vi "JKI_DataBase.vi"() -> ()   [LabVIEW 2017, in "Database.lvlib"]
uses:
  Database.lvlib
  <userlib>/_NEVSTOP/JKI State Machine ++/_Support/_Create Data Queue.vi
  <vilib>/Utility/file.llb/Read Delimited Spreadsheet (string).vi
  <userlib>/_NEVSTOP/JKI State Machine ++/_Support/_JKISMQFGV.vi
  <vilib>/Utility/file.llb/Write Delimited Spreadsheet (string).vi
  <userlib>/_NEVSTOP/JKI State Machine ++/JKI-State-Machine-Plus.lvlib
panel:
  in  "Error Simulator":bool
  out "Balance":i32
  out "Find Account?":bool
  in  "Get Balance Simulator":bool
  in  "Update Simulator":bool
  in  "Find Account Simulator":bool
  out "若有需要返回用户姓名，后面也可以接到esponse上":string
  out "State History":string
  in  "Name(\"\" to use uuid)":string="Database"
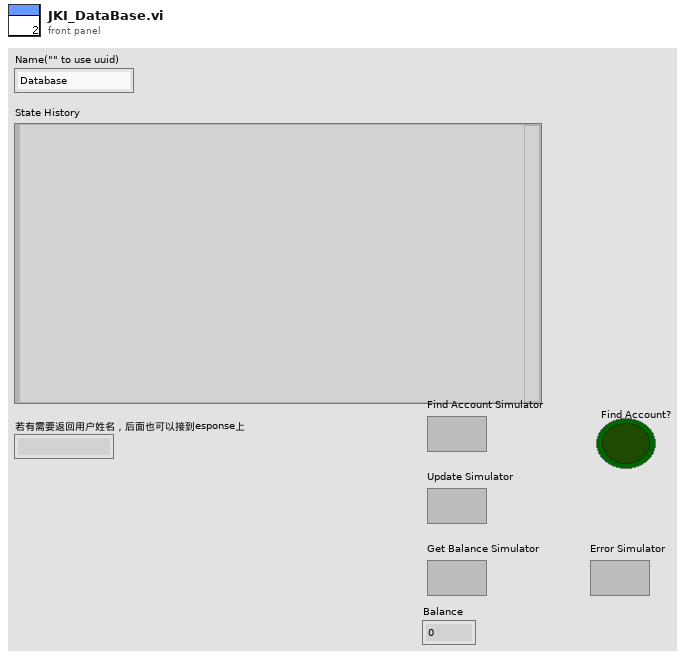
[diagram p1: front panel]
types:
  T1 = enum32{"Invalid", "Standard", "Closed", "Hidden", "Minimized", "Maximized"}
  T2 = enum32{"invalid app kind", "Development System", "Run Time System", "Student Edition", "Embedded LabVIEW", "Evaluation", "Custom"}
  T3 = cluster{"Core":cluster{"Current VI Reference":refnum<vi>, "Close Panel on Exit?":bool}}
  T4 = cluster{"PIN":string, "First":string, "Last":string, "Amount":string}
  T5 = cluster{"Current VI Reference":refnum<vi>, "Close Panel on Exit?":bool}
  T6 = cluster{"PIN":string, "First":string, "Last":string, "Amount":string}[]
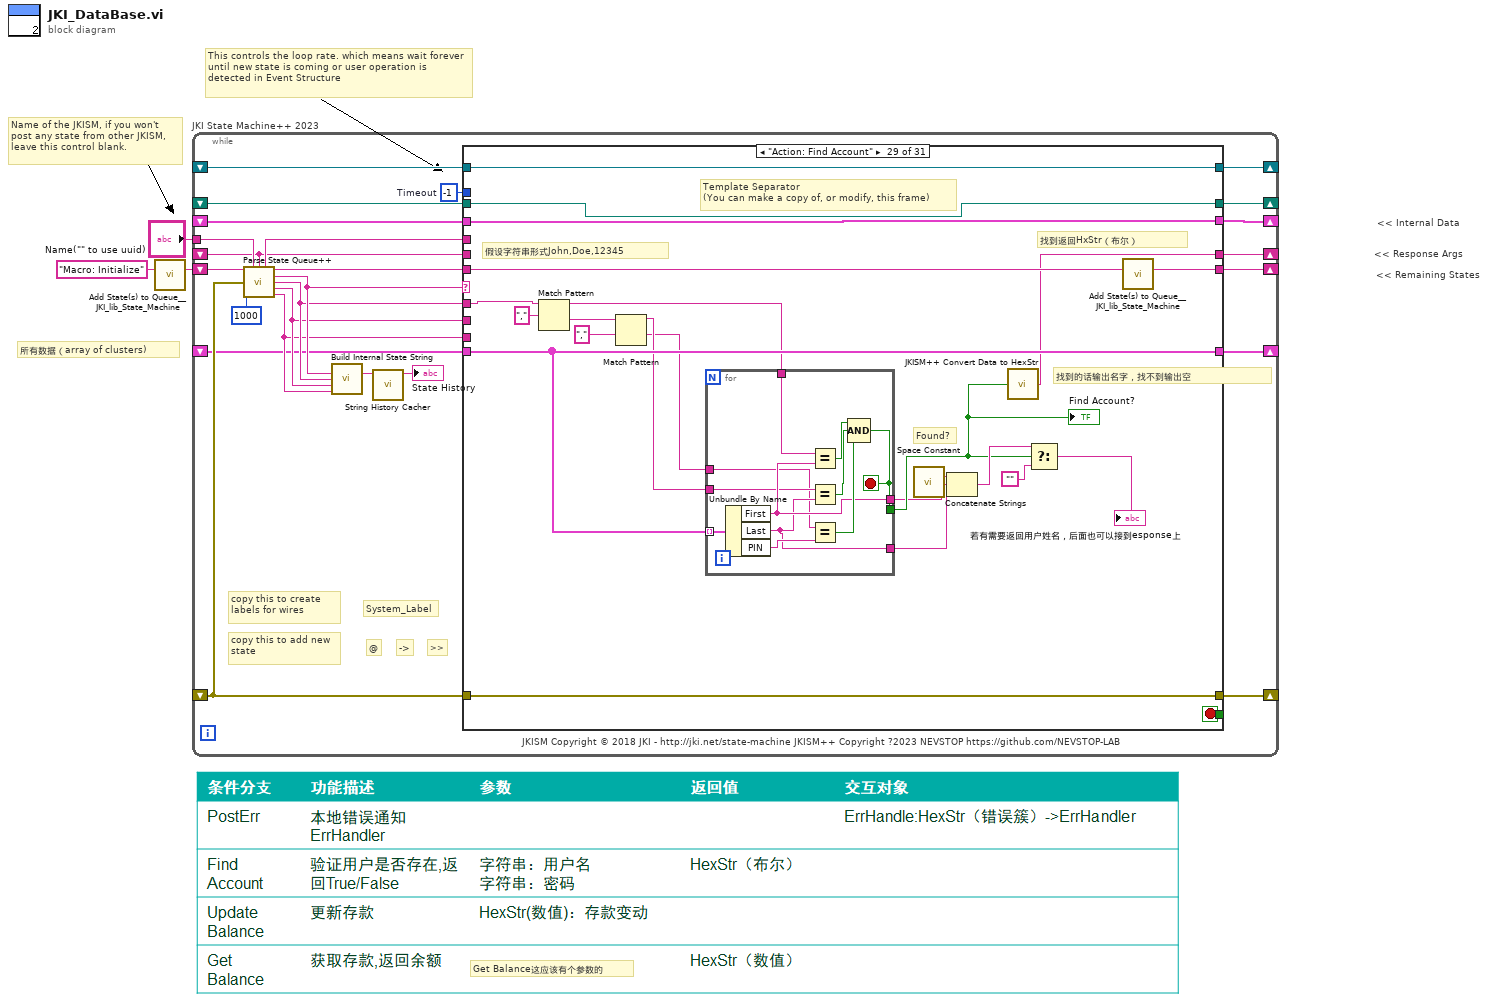
[diagram p0: block diagram]
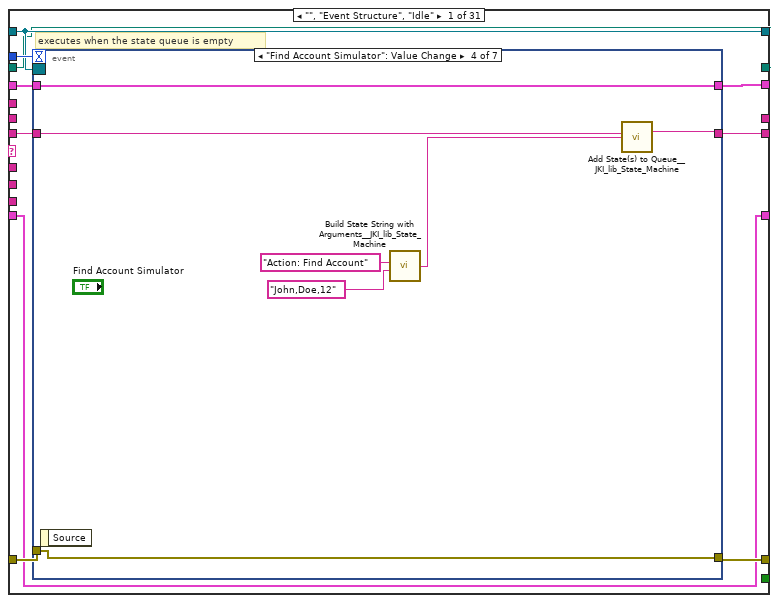
[diagram p2: hidden frame]
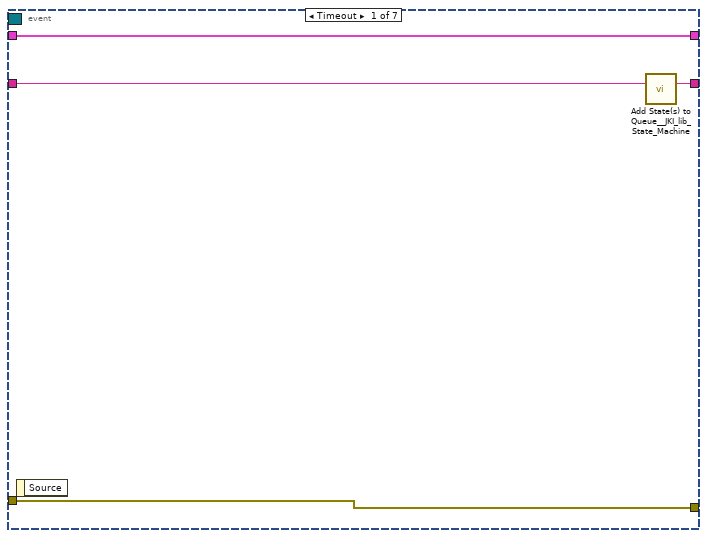
[diagram p3: hidden frame]
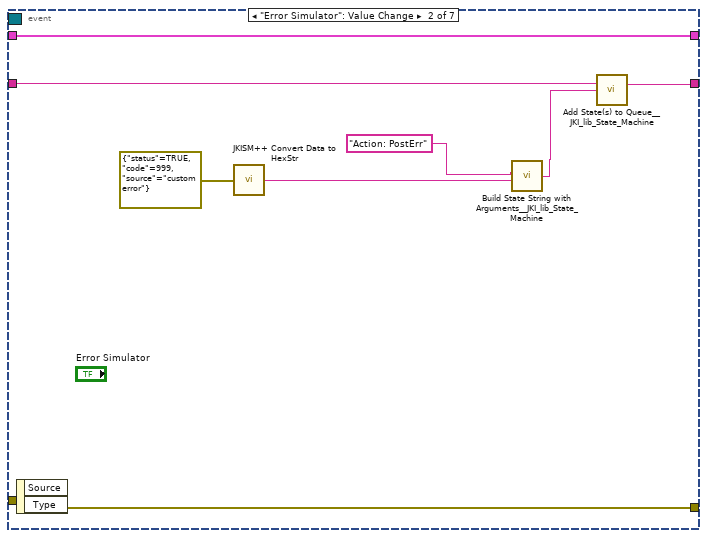
[diagram p4: hidden frame]
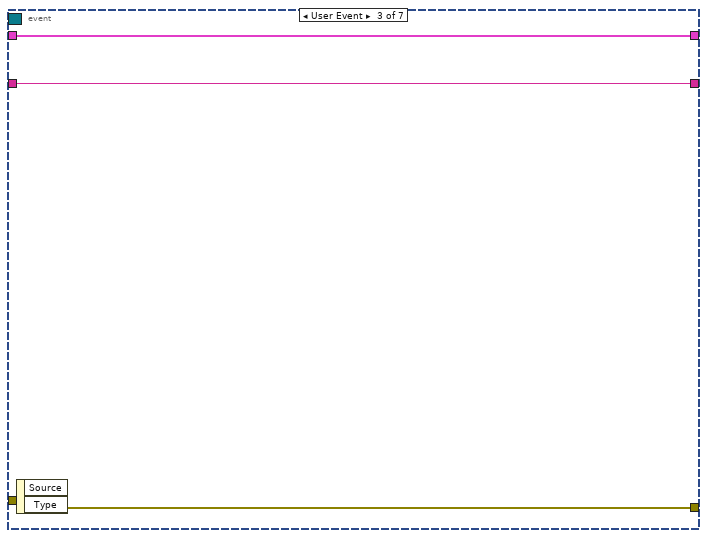
[diagram p5: hidden frame]
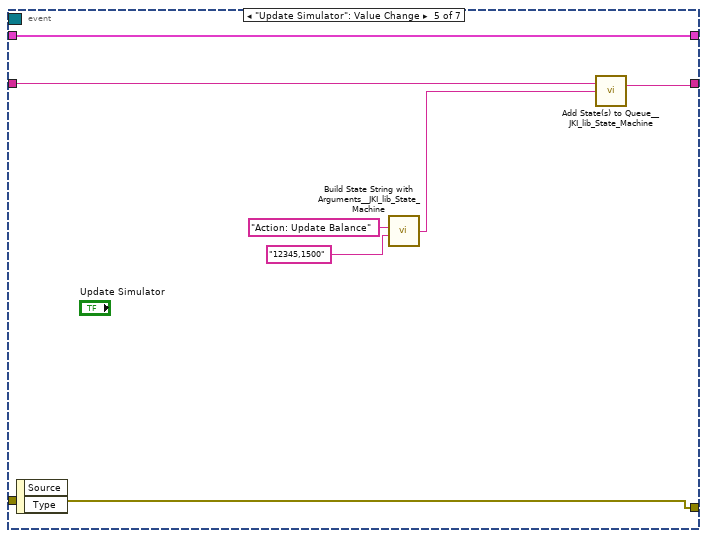
[diagram p6: hidden frame]
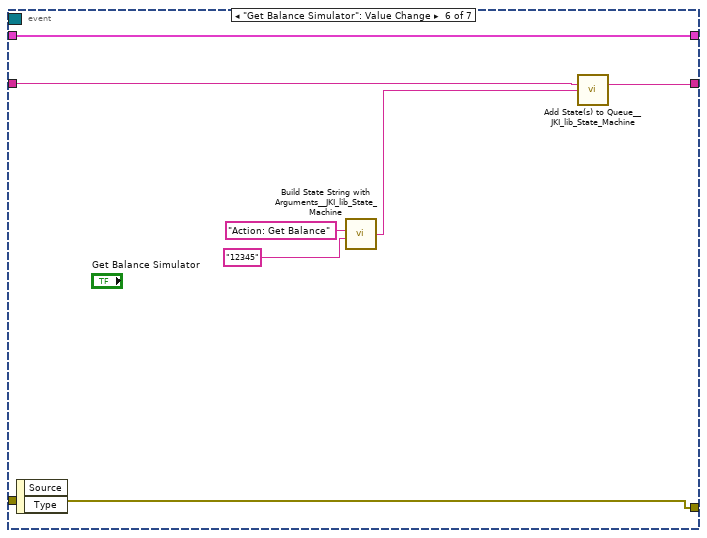
[diagram p7: hidden frame]
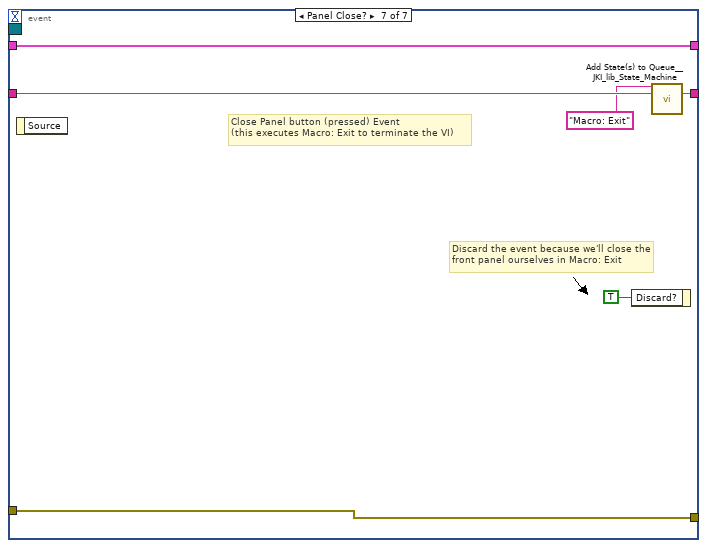
[diagram p8: hidden frame]
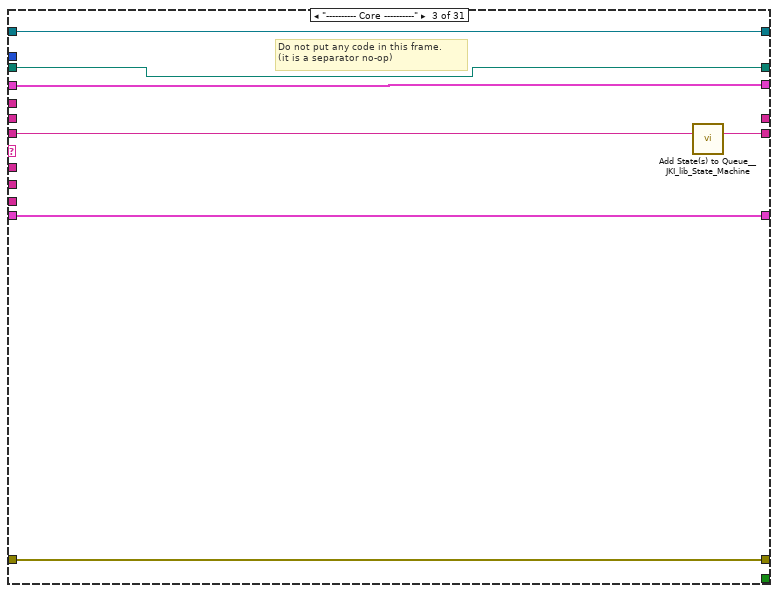
[diagram p10: hidden frame]
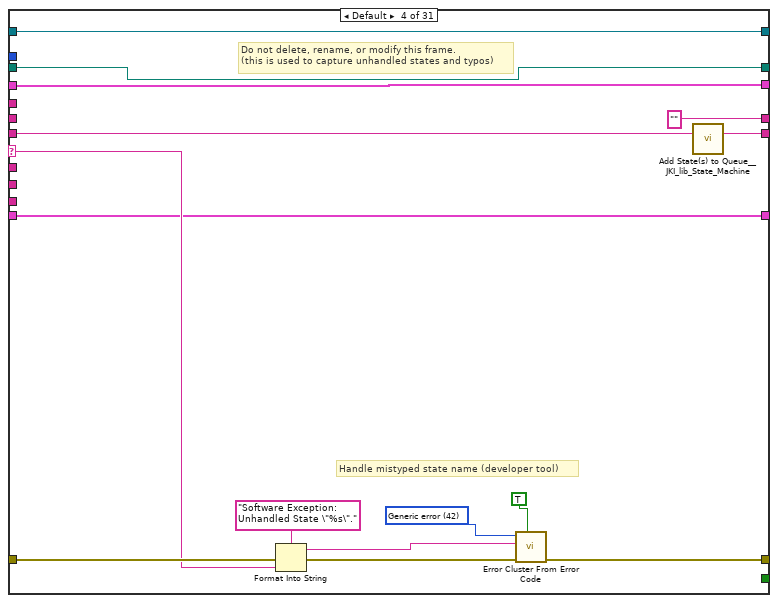
[diagram p11: hidden frame]
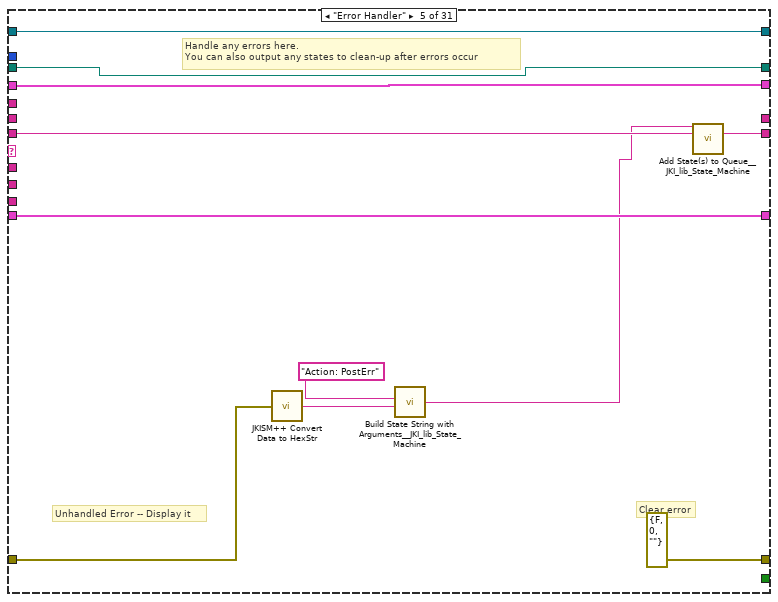
[diagram p12: hidden frame]
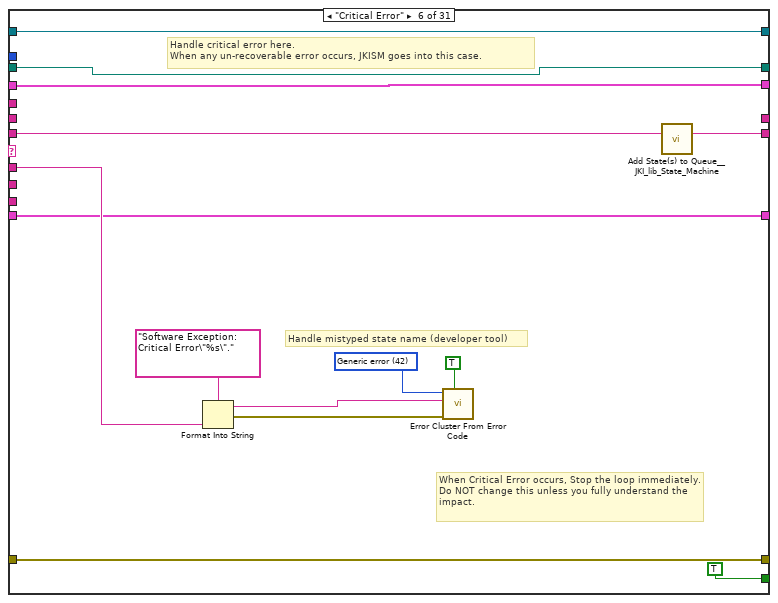
[diagram p13: hidden frame]
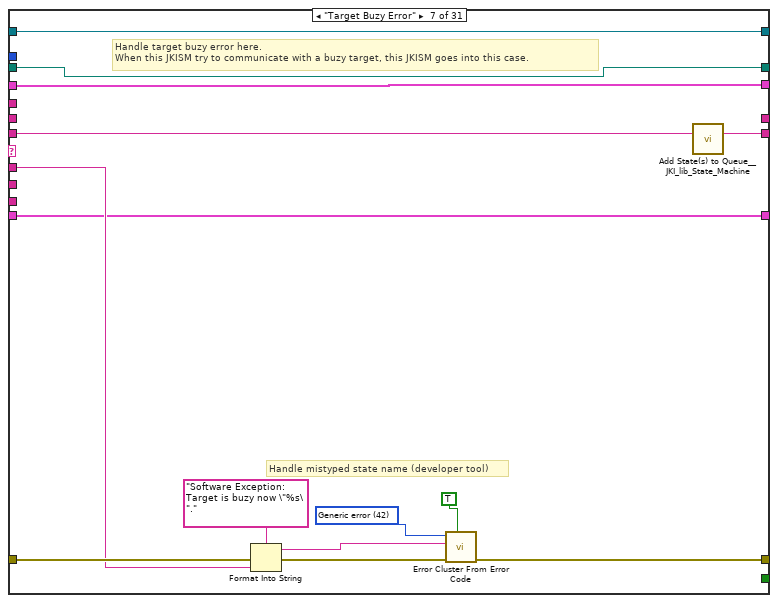
[diagram p14: hidden frame]
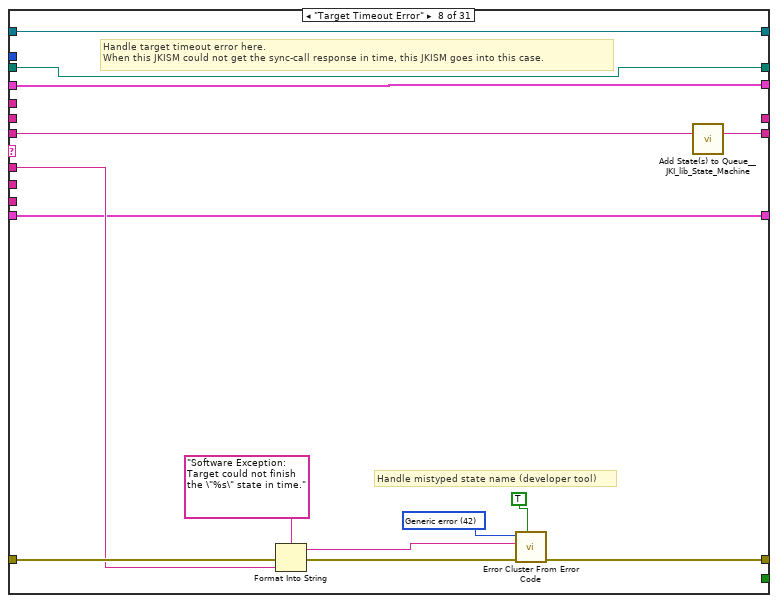
[diagram p15: hidden frame]
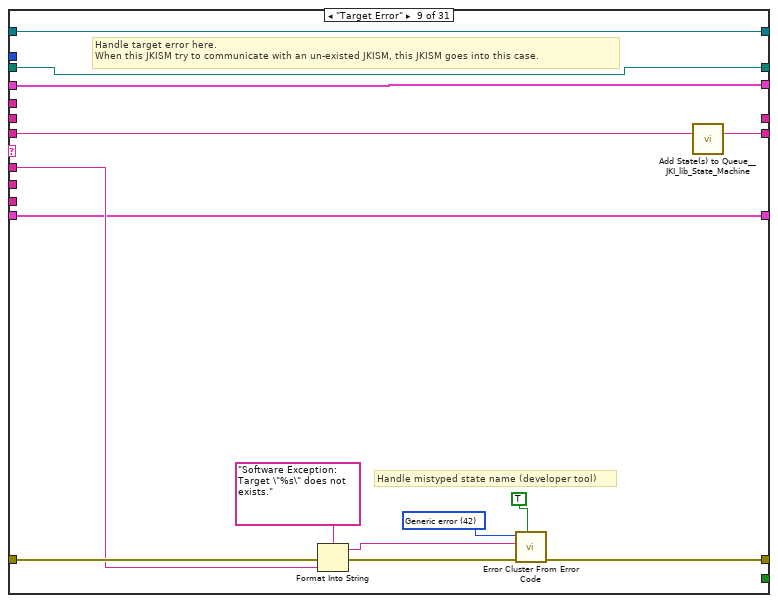
[diagram p16: hidden frame]
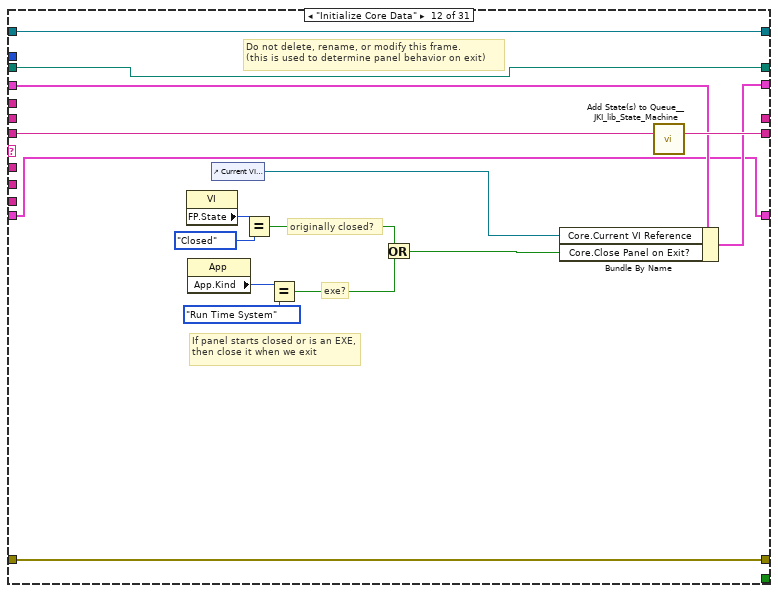
[diagram p19: hidden frame]
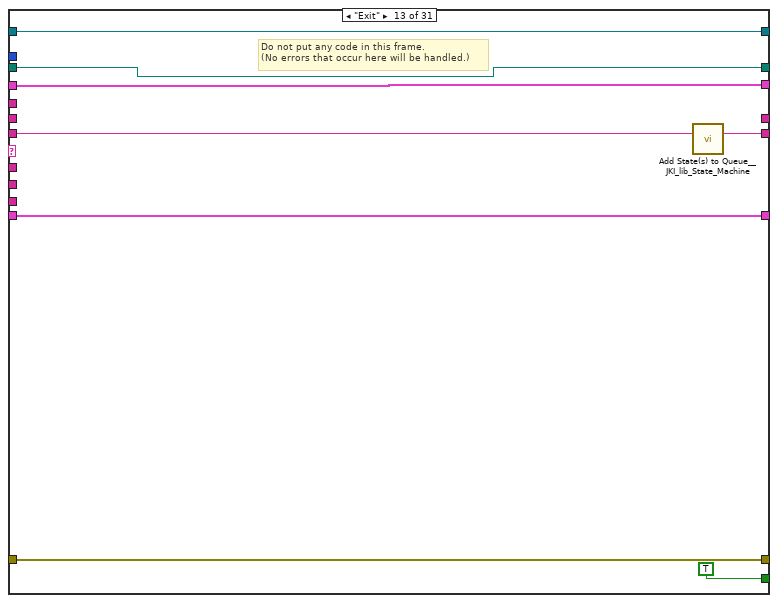
[diagram p20: hidden frame]
diagram:
  # "Get Balance这应该有个参数的"
  # "所有数据（array of clusters)"
  # "<< Internal Data"
  # "<< Response Args"
  # "<< Remaining States"
  # "Name of the JKISM, if you won't post any state from other JKISM,  leave this control blank."
  # "This controls the loop rate. which means wait forever until new state is coming or user operation is detected in Event Structure"
  n1 = call <vilib>:"Add State(s) to Queue__JKI_lib_State_Machine.vi"("State(s) in (\"\")"="Macro: Initialize") -> ("States Out"=w1:string)  [unwired: 14 in]
  n2 = while "JKI State Machine++ 2023" {
    shift-right: [w24] -> _
    shift-left: _ -> [w23]
    shift-right: [w27] -> _
    shift-left: _ -> [w21]
    shift-right: [w26] -> _
    shift-left: w1 -> [w28]
    tunnel: "Name(\"\" to use uuid)" -> [w16]
    shift-right: [w19] -> _
    shift-left: _ -> [w8]
    shift-right: [w18] -> _
    shift-left: _ -> [w17]
    shift-right: [w7] -> _
    shift-left: _ -> [w6]
    shift-right: [w5] -> _
    shift-left: _ -> [w4]
    stop <- w25 stop-if-true
    w22 = -1  # Timeout
    # "JKISM Copyright © 2018 JKI - http://jki.net/state-machine JKISM++ Copyright ?2023 NEVSTOP https://github.com/NEVSTOP-LAB"
    # "copy this to add new state"
    # ">>"
    # "->"
    # "@"
    # "copy this to create labels for wires"
    # "System_Label"
    n3 = call <userlib>:"Parse State Queue++.vi"("State Queue"=w28, "Name(\"\" to use uuid)"=w16, "Response Arguments"=w8, "Error In (no error)"=w21, "Response Timeout(5000ms)"=1000 ("Response Timeout(1000ms)")) -> ("Name Used"=w9:string, "Remaining States"=w29:string, "Current State"=w13:string, "Arguments"=w12:string, "Argument - State"=w11:string, "From Who"=w10:string)  [unwired: 5 in]
    n4 = call <userlib>:"Build Internal State String.vi"("State"=w13, "Arguments (\"\")"=w12, "Arg-State (\"\")"=w11, "Source (\"\")"=w10) -> ("State with Arguments"=w14:string)  [unwired: 11 in]
    n5 = call <userlib>:"String History Cacher.vi"("String"=w14) -> ("String Cache"=→"State History":string)  [unwired: 10 in]
    n6 = case shown="\"Action: Find Account\"" w13 {
      selector: w13 -> [_ _ _ w99 _ _ _ _ _ _ _ _ _ _ _ _ _ _ _ _ _ _ _ _ _ _ _ _ _ _ _]
      tunnel: w29 -> [w39 w86 w94 w103 w120 w132 w137 w156 w170 w181 w187 w204 w212 w219 w232 w248 w255 w263 w269 w277 w284 w293 w307 w374 w382 w395 w402 w410 w435 w474 w492]
      tunnel: w12 -> [_ _ _ _ _ w125 w139 w152 w166 _ _ _ _ _ _ _ _ _ _ _ _ w288 w302 _ _ _ _ w406 w428 w460 w485]
      tunnel: w23 -> [w37 w85 w91 w101 w117 w133 w141 w154 w168 w180 w186 w191 w210 w216 _ w242 w252 w262 w268 w274 w282 w291 w299 w371 w379 w385 w399 w414 w434 w472 w489]
      tunnel: [w36 w87 w92 w105 errorcluster {"status"=FALSE, "code"=0, "source"=""} ("error out") w134 w144 w158 w172 w182 w188 w202 w209 w217 w230 w245 w253 w258 w267 w275 w281 w289 w304 w372 w380 w393 w400 w404 w445 w461 w490] -> w27
      tunnel: w21 -> [w35 w87 w92 w104 w111 w134 w143 w157 w171 w182 w188 w202 w209 w217 w230 w246 w253 _ w270 w275 w281 w290 w305 w372 w380 w393 w400 w405 w445 _ w490]
      tunnel: [w38 w86 w93 w102 w119 w131 w142 w155 w169 w181 w187 w203 w211 w218 w231 w247 w254 w263 w269 w276 w283 w292 w306 w373 w381 w394 w401 w409 w436 w473 w491] -> w26
      tunnel: [_ _ _ _ _ TRUE _ _ _ _ _ _ TRUE _ _ _ _ _ _ _ _ _ _ _ _ _ _ _ _ _ _] -> w25
      tunnel: [w34 w85 w91 w101 w117 w133 w141 w154 w168 w180 w186 w190 w210 w216 w221 w242 w252 w262 w268 w274 w282 w291 w299 w371 w379 w385 w399 w414 w434 w472 w489] -> w24
      tunnel: w22 -> [w33 _ _ _ _ _ _ _ _ _ _ _ _ _ _ _ _ _ _ _ _ _ _ _ _ _ _ _ _ _ _]
      tunnel: w10 -> [_ _ _ _ _ _ _ _ _ _ _ _ _ _ _ _ _ _ _ _ _ _ _ _ _ _ _ _ _ _ _]
      tunnel: w11 -> [_ _ _ _ _ _ _ _ _ _ _ _ _ _ _ _ _ _ _ _ _ _ _ _ _ _ _ _ _ _ _]
      tunnel: [_ _ _ "" _ _ _ _ _ _ _ _ _ _ _ _ _ _ _ _ _ _ _ _ _ _ _ _ w424 _ w483] -> w19
      tunnel: [w32 w84 w90 w97 w116 w123 w138 w151 w165 w179 w185 w193 w207 w215 w228 w244 w251 w261 w266 w273 w280 w287 w301 w370 w377 w387 w398 w413 w444 w471 w488] -> w18
      tunnel: w17 -> [w32 w84 w90 w97 w116 w123 w138 w151 w165 w179 w185 w193 w207 w215 w228 w244 w251 _ w266 w273 w280 w287 w301 w370 w377 w387 w398 w413 w444 w471 w488]
      tunnel: w9 -> [_ _ _ _ _ _ _ _ _ _ _ _ _ _ _ _ _ w260 _ _ _ _ _ _ _ _ _ _ _ _ _]
      tunnel: w8 -> [_ _ _ _ _ _ _ _ _ _ _ _ _ _ _ _ _ _ _ _ _ _ _ _ _ _ _ _ _ _ _]
      tunnel: [w31 w83 w89 w96 w115 w122 w136 w150 w164 w178 w184 w192 w206 w214 w223 w243 w250 w257 w265 w272 w279 w286 w300 w369 w376 w386 w397 w412 w443 w463 w487] -> w7
      tunnel: w6 -> [w31 w83 w89 w96 w115 w122 w136 w150 w164 w178 w184 w192 w206 w214 _ w243 w250 w257 w265 w272 w279 w286 w300 w369 w376 w386 w397 w412 w443 w463 w487]
      tunnel: [w30 w82 w88 w95 w114 w121 w135 w149 w163 w177 w183 w189 w205 w213 w220 w240 w249 w256 w264 w271 w278 w285 w298 w368 w375 w383 w396 w411 w439 w462 w486] -> w5
      tunnel: w4 -> [w30 w82 w88 w95 w114 w121 w135 w149 w163 w177 w183 w189 w205 w213 _ w240 w249 w256 w264 w271 w278 w285 w298 w368 w375 w383 w396 w411 w439 w468 w486]
      frame "", "Event Structure", "Idle" {
        # "executes when the state queue is empty"
        n7 = event shown="[3] \"Find Account Simulator\": Value Change" {
          selector: w32 -> [_ _ _ _ _ _ _]
          dyn-events: _ -> [_ _ _ _ _ _ _]
          timeout: w33 -> [_ _ _ _ _ _ _]
          tunnel: w39 -> [w43 w46 w54 w59 w66 w71 w81]
          tunnel: [w42 w45 w54 w58 w65 w70 w80] -> w38
          tunnel: w37 -> [w40 w50 w52 w61 w68 w75 w78]
          tunnel: [w41 w51 w53 w60 w67 w74 w79] -> w36
          tunnel: w35 -> [w41 w51 w53 w60 w67 w74 w79]
          tunnel: [w40 w50 w52 w61 w68 w75 w78] -> w34
          event Timeout {
            n8 = event-data() -> ()  [unwired: 1 in, 1 out]
            n9 = call <vilib>:"Add State(s) to Queue__JKI_lib_State_Machine.vi"("State(s) in (\"\")"=w43) -> ("States Out"=w42:string)  [unwired: 14 in]
          }
          event "Error Simulator": Value Change {
            n10 = event-data() -> ()  [unwired: 1 in, 2 out]
            n11 = call <userlib>:"JKISM++ Convert Data to HexStr.vi"("Variant"=errorcluster {"status"=TRUE, "code"=999, "source"="custom error"} ("error in (no error)")) -> ("HEX String (0-9,A-F)"=w47:string)  [unwired: 8 in]
            n12 = call <vilib>:"Build State String with Arguments__JKI_lib_State_Machine.vi"("Arguments (\"\")"=w47, "State"="Action: PostErr" ("States")) -> ("State with Arguments"=w44:string)  [unwired: 4 in]
            n13 = call <vilib>:"Add State(s) to Queue__JKI_lib_State_Machine.vi"("State(s) in (\"\")"=w46, "State(s) at Back (\"\")"=w44) -> ("States Out"=w45:string)  [unwired: 13 in]
          }
          event User Event {
            n14 = event-data() -> ()  [unwired: 1 in, 2 out]
          }
          event "Find Account Simulator": Value Change {
            n15 = event-data() -> ()  [unwired: 1 in, 1 out]
            n16 = call <vilib>:"Build State String with Arguments__JKI_lib_State_Machine.vi"("Arguments (\"\")"="John,Doe,12", "State"="Action: Find Account") -> ("State with Arguments"=w55:string)  [unwired: 4 in]
            n17 = call <vilib>:"Add State(s) to Queue__JKI_lib_State_Machine.vi"("State(s) in (\"\")"=w59, "State(s) at Back (\"\")"=w55) -> ("States Out"=w58:string)  [unwired: 13 in]
          }
          event "Update Simulator": Value Change {
            n18 = event-data() -> ()  [unwired: 1 in, 2 out]
            n19 = call <vilib>:"Build State String with Arguments__JKI_lib_State_Machine.vi"("Arguments (\"\")"="12345,1500", "State"="Action: Update Balance") -> ("State with Arguments"=w62:string)  [unwired: 4 in]
            n20 = call <vilib>:"Add State(s) to Queue__JKI_lib_State_Machine.vi"("State(s) in (\"\")"=w66, "State(s) at Back (\"\")"=w62) -> ("States Out"=w65:string)  [unwired: 13 in]
          }
          event "Get Balance Simulator": Value Change {
            n21 = event-data() -> ()  [unwired: 1 in, 2 out]
            n22 = call <vilib>:"Build State String with Arguments__JKI_lib_State_Machine.vi"("Arguments (\"\")"="12345", "State"="Action: Get Balance") -> ("State with Arguments"=w69:string)  [unwired: 4 in]
            n23 = call <vilib>:"Add State(s) to Queue__JKI_lib_State_Machine.vi"("State(s) in (\"\")"=w71, "State(s) at Back (\"\")"=w69) -> ("States Out"=w70:string)  [unwired: 13 in]
          }
          event Panel Close? {
            # "Discard the event because we'll close the front panel ourselves in Macro: Exit"
            # "Close Panel button (pressed) Event\n(this executes Macro: Exit to terminate the VI)"
            n24 = event-data() -> ()  [unwired: 1 in, 1 out]
            n25 = event-data("Discard?"=TRUE) -> ()  [unwired: 1 in, 1 out]
            n26 = call <vilib>:"Add State(s) to Queue__JKI_lib_State_Machine.vi"("State(s) in Front (\"\")"="Macro: Exit", "State(s) in (\"\")"=w81) -> ("States Out"=w80:string)  [unwired: 13 in]
          }
        }
      }
      frame "JKISM++ Documentation" {
        # "JKISM++ Documentation"
        # "State Syntax:\nStateCategory: State >> Argument @|-> JKISMName\nLine Terminator: Line feed\n\nExample:\nUI: Help >> About @Main\nUI: Help >> About ->Main"
        # "Commenting:\nTo add a comment use \"//\" or \"#\" and all text to the right will be ignored\nCommenting Example:\nUI: Initialize // This initializes the UI\n# This whole line is a comment\n// Another comment line"
        # "Where \"UI\" is the state category\nWhere \"Help\" is the state\nWhere \"About\" is the argument\nWhere \"Main\" is the Name of JKISM,which actually run the \"UI: Help >> About\"\n\n    \"@\" stands for sync state. Current JKISM will wait until the state is finished. \n            - if \"Main\" named JKISM does not exist, \"Target Error\" will occur.\n            - if \"Main\" named JKISM is in another sync remote state, \"Target Buzy Error\" will occur.\n            - if \"Main\" named JKISM could not finish the state in time, \"Target Timeout Error\" will occur.\n            - if everything is right. \"Response\" will occur with Argument back from \"Main\" named JKISM. \n\n    \"->\" stands for async state. Current JKISM will post the state and continue to next state in next iteration.\n            - if \"Main\" named JKISM does not exist, \"Target Error\" will occur.\n            - if everything is right. \"Async Message Posted\" will occur.\n            - After State is finished. Caller will receive a \"Async Response\" state from callee.\n\nWhen duplicated name is used for multiple JKISM module or some framework problem happens, \"Critical Error\" will occur."
      }
      frame "---------- Core ----------" {
        # "Do not put any code in this frame.\n(it is a separator no-op)"
        n27 = call <vilib>:"Add State(s) to Queue__JKI_lib_State_Machine.vi"("State(s) in (\"\")"=w94) -> ("States Out"=w93:string)  [unwired: 14 in]
      }
      frame Default {
        w108 = 42 items=["No error", "Argument error", "Memory is full", "Out of zone", "End of file", "File already open", "Generic file I/O error", "File not found", "File permission error", "Disk is full", "Duplicate path", "Too many files open", "System feature not enabled", "Resource file not found", "Cannot add resource", "Resource not found", "Image not found", "Image memory error", "Pen does not exist", "Config type invalid", "Config token not found", "Config parse error", "Config memory error", "Bad external code format", "Bad external code offset", "External code not present", "Null window", "Destroy window error", "Null menu", "Print aborted", "Bad print record", "Print driver error", "Windows error during printing", "Memory error during printing", "Print dialog error", "Generic print error", "Invalid device refnum", "Device not found", "Device parameter error", "Device unit error", "Cannot open device", "Device call aborted", "Generic error", "Cancelled by user", "Object ID too low", "Object ID too high", "Object not in heap", "Unknown heap", "Unknown object (invalid DefProc)", "Unknown object (DefProc not in table)", "Message out of range", "Invalid (null) method", "Unknown message", "Manager call not supported", "Bad address", "Network operation in progress", "Network operation timed out", "Connection is busy", "Network attribute not supported", "Network error", "Address in use", "System out of memory", "Connection aborted", "Connection refused", "Not connected", "Already connected", "Connection closed", "Initialization error (interapplication manager)", "Bad occurrence", "Wait on unbound occurrence handler", "Occurrence queue overflow", "Datalog type conflict", "Unused", "Unrecognized type (interapplication manager)", "Memory corrupt", "Failed to make temporary DLL", "Old CIN version", "Drag socket not found", "Failed to load drop-object", "Failed to register OLE object", "Failed to release OLE object", "Format specifier type mismatch", "Unknown format specifier", "Too few format specifiers", "Too many format specifiers", "Scan failed", "Newer CIN version", "Error converting to variant", "Runtime menu error", "Password tampered", "Variant attribute not found", "Incompatible variant data type", "Event data is not available", "Event Store is not present", "Occurrence is not found", "Event Queue is not created", "Event info is not available", "Refnum passed is NULL", "Error retrieving Class GUID", "Error retrieving CoClass GUID", "Error retrieving TypeLib GUID.", "Bad built application magic bytes.", "Specific driver is different from the specific driver associated with the Logical Name.", "There is no session opened to the class driver.", "Max Error", "MAX - Error with config objects", "MAX - Error loading configuration", "MAX - Group not supported"]
        # "Do not delete, rename, or modify this frame.\n(this is used to capture unhandled states and typos)"
        # "Handle mistyped state name (developer tool)"
        n28 = Format Into String(format string="Software Exception: Unhandled State \"%s\"." ("message"), error in=w104, w99) -> (resulting string=w107:string, error out=w106:errorcluster)  [unwired: 1 in]
        n29 = call <vilib>:"Error Cluster From Error Code.vi"("show call chain? (False)"=TRUE, "error in (no error)"=w106, "error message (\"\")"=w107, "error code (0)"=w108) -> ("error out"=w105:errorcluster)  [unwired: 5 in]
        n30 = call <vilib>:"Add State(s) to Queue__JKI_lib_State_Machine.vi"("State(s) in (\"\")"=w103) -> ("States Out"=w102:string)  [unwired: 14 in]
      }
      frame "Error Handler" {
        # "Unhandled Error -- Display it"
        # "Handle any errors here.\nYou can also output any states to clean-up after errors occur"
        # "Clear error"
        n31 = call <userlib>:"JKISM++ Convert Data to HexStr.vi"("Variant"=w111) -> ("HEX String (0-9,A-F)"=w113:string)  [unwired: 8 in]
        n32 = call <vilib>:"Build State String with Arguments__JKI_lib_State_Machine.vi"("Arguments (\"\")"=w113, "State"="Action: PostErr") -> ("State with Arguments"=w110:string)  [unwired: 4 in]
        n33 = call <vilib>:"Add State(s) to Queue__JKI_lib_State_Machine.vi"("State(s) in Front (\"\")"=w110, "State(s) in (\"\")"=w120) -> ("States Out"=w119:string)  [unwired: 13 in]
      }
      frame "Critical Error" {
        w129 = 42 items=["No error", "Argument error", "Memory is full", "Out of zone", "End of file", "File already open", "Generic file I/O error", "File not found", "File permission error", "Disk is full", "Duplicate path", "Too many files open", "System feature not enabled", "Resource file not found", "Cannot add resource", "Resource not found", "Image not found", "Image memory error", "Pen does not exist", "Config type invalid", "Config token not found", "Config parse error", "Config memory error", "Bad external code format", "Bad external code offset", "External code not present", "Null window", "Destroy window error", "Null menu", "Print aborted", "Bad print record", "Print driver error", "Windows error during printing", "Memory error during printing", "Print dialog error", "Generic print error", "Invalid device refnum", "Device not found", "Device parameter error", "Device unit error", "Cannot open device", "Device call aborted", "Generic error", "Cancelled by user", "Object ID too low", "Object ID too high", "Object not in heap", "Unknown heap", "Unknown object (invalid DefProc)", "Unknown object (DefProc not in table)", "Message out of range", "Invalid (null) method", "Unknown message", "Manager call not supported", "Bad address", "Network operation in progress", "Network operation timed out", "Connection is busy", "Network attribute not supported", "Network error", "Address in use", "System out of memory", "Connection aborted", "Connection refused", "Not connected", "Already connected", "Connection closed", "Initialization error (interapplication manager)", "Bad occurrence", "Wait on unbound occurrence handler", "Occurrence queue overflow", "Datalog type conflict", "Unused", "Unrecognized type (interapplication manager)", "Memory corrupt", "Failed to make temporary DLL", "Old CIN version", "Drag socket not found", "Failed to load drop-object", "Failed to register OLE object", "Failed to release OLE object", "Format specifier type mismatch", "Unknown format specifier", "Too few format specifiers", "Too many format specifiers", "Scan failed", "Newer CIN version", "Error converting to variant", "Runtime menu error", "Password tampered", "Variant attribute not found", "Incompatible variant data type", "Event data is not available", "Event Store is not present", "Occurrence is not found", "Event Queue is not created", "Event info is not available", "Refnum passed is NULL", "Error retrieving Class GUID", "Error retrieving CoClass GUID", "Error retrieving TypeLib GUID.", "Bad built application magic bytes.", "Specific driver is different from the specific driver associated with the Logical Name.", "There is no session opened to the class driver.", "Max Error", "MAX - Error with config objects", "MAX - Error loading configuration", "MAX - Group not supported"]
        # "Handle critical error here.\nWhen any un-recoverable error occurs, JKISM goes into this case."
        # "When Critical Error occurs, Stop the loop immediately. Do NOT change this unless you fully understand the impact."
        # "Handle mistyped state name (developer tool)"
        n34 = Format Into String(format string="Software Exception: Critical Error\"%s\"." ("message"), w125) -> (resulting string=w128:string, error out=w127:errorcluster)  [unwired: 2 in]
        n35 = call <vilib>:"Error Cluster From Error Code.vi"("show call chain? (False)"=TRUE, "error in (no error)"=w127, "error message (\"\")"=w128, "error code (0)"=w129) -> ()  [unwired: 5 in, 1 out]
        n36 = call <vilib>:"Add State(s) to Queue__JKI_lib_State_Machine.vi"("State(s) in (\"\")"=w132) -> ("States Out"=w131:string)  [unwired: 14 in]
      }
      frame "Target Buzy Error" {
        w147 = 42 items=["No error", "Argument error", "Memory is full", "Out of zone", "End of file", "File already open", "Generic file I/O error", "File not found", "File permission error", "Disk is full", "Duplicate path", "Too many files open", "System feature not enabled", "Resource file not found", "Cannot add resource", "Resource not found", "Image not found", "Image memory error", "Pen does not exist", "Config type invalid", "Config token not found", "Config parse error", "Config memory error", "Bad external code format", "Bad external code offset", "External code not present", "Null window", "Destroy window error", "Null menu", "Print aborted", "Bad print record", "Print driver error", "Windows error during printing", "Memory error during printing", "Print dialog error", "Generic print error", "Invalid device refnum", "Device not found", "Device parameter error", "Device unit error", "Cannot open device", "Device call aborted", "Generic error", "Cancelled by user", "Object ID too low", "Object ID too high", "Object not in heap", "Unknown heap", "Unknown object (invalid DefProc)", "Unknown object (DefProc not in table)", "Message out of range", "Invalid (null) method", "Unknown message", "Manager call not supported", "Bad address", "Network operation in progress", "Network operation timed out", "Connection is busy", "Network attribute not supported", "Network error", "Address in use", "System out of memory", "Connection aborted", "Connection refused", "Not connected", "Already connected", "Connection closed", "Initialization error (interapplication manager)", "Bad occurrence", "Wait on unbound occurrence handler", "Occurrence queue overflow", "Datalog type conflict", "Unused", "Unrecognized type (interapplication manager)", "Memory corrupt", "Failed to make temporary DLL", "Old CIN version", "Drag socket not found", "Failed to load drop-object", "Failed to register OLE object", "Failed to release OLE object", "Format specifier type mismatch", "Unknown format specifier", "Too few format specifiers", "Too many format specifiers", "Scan failed", "Newer CIN version", "Error converting to variant", "Runtime menu error", "Password tampered", "Variant attribute not found", "Incompatible variant data type", "Event data is not available", "Event Store is not present", "Occurrence is not found", "Event Queue is not created", "Event info is not available", "Refnum passed is NULL", "Error retrieving Class GUID", "Error retrieving CoClass GUID", "Error retrieving TypeLib GUID.", "Bad built application magic bytes.", "Specific driver is different from the specific driver associated with the Logical Name.", "There is no session opened to the class driver.", "Max Error", "MAX - Error with config objects", "MAX - Error loading configuration", "MAX - Group not supported"]
        # "Handle target buzy error here.\nWhen this JKISM try to communicate with a buzy target, this JKISM goes into this case."
        # "Handle mistyped state name (developer tool)"
        n37 = Format Into String(format string="Software Exception: Target is buzy now \"%s\"." ("message"), error in=w143, w139) -> (resulting string=w146:string, error out=w145:errorcluster)  [unwired: 1 in]
        n38 = call <vilib>:"Error Cluster From Error Code.vi"("show call chain? (False)"=TRUE, "error in (no error)"=w145, "error message (\"\")"=w146, "error code (0)"=w147) -> ("error out"=w144:errorcluster)  [unwired: 5 in]
        n39 = call <vilib>:"Add State(s) to Queue__JKI_lib_State_Machine.vi"("State(s) in (\"\")"=w137) -> ("States Out"=w142:string)  [unwired: 14 in]
      }
      frame "Target Timeout Error" {
        w161 = 42 items=["No error", "Argument error", "Memory is full", "Out of zone", "End of file", "File already open", "Generic file I/O error", "File not found", "File permission error", "Disk is full", "Duplicate path", "Too many files open", "System feature not enabled", "Resource file not found", "Cannot add resource", "Resource not found", "Image not found", "Image memory error", "Pen does not exist", "Config type invalid", "Config token not found", "Config parse error", "Config memory error", "Bad external code format", "Bad external code offset", "External code not present", "Null window", "Destroy window error", "Null menu", "Print aborted", "Bad print record", "Print driver error", "Windows error during printing", "Memory error during printing", "Print dialog error", "Generic print error", "Invalid device refnum", "Device not found", "Device parameter error", "Device unit error", "Cannot open device", "Device call aborted", "Generic error", "Cancelled by user", "Object ID too low", "Object ID too high", "Object not in heap", "Unknown heap", "Unknown object (invalid DefProc)", "Unknown object (DefProc not in table)", "Message out of range", "Invalid (null) method", "Unknown message", "Manager call not supported", "Bad address", "Network operation in progress", "Network operation timed out", "Connection is busy", "Network attribute not supported", "Network error", "Address in use", "System out of memory", "Connection aborted", "Connection refused", "Not connected", "Already connected", "Connection closed", "Initialization error (interapplication manager)", "Bad occurrence", "Wait on unbound occurrence handler", "Occurrence queue overflow", "Datalog type conflict", "Unused", "Unrecognized type (interapplication manager)", "Memory corrupt", "Failed to make temporary DLL", "Old CIN version", "Drag socket not found", "Failed to load drop-object", "Failed to register OLE object", "Failed to release OLE object", "Format specifier type mismatch", "Unknown format specifier", "Too few format specifiers", "Too many format specifiers", "Scan failed", "Newer CIN version", "Error converting to variant", "Runtime menu error", "Password tampered", "Variant attribute not found", "Incompatible variant data type", "Event data is not available", "Event Store is not present", "Occurrence is not found", "Event Queue is not created", "Event info is not available", "Refnum passed is NULL", "Error retrieving Class GUID", "Error retrieving CoClass GUID", "Error retrieving TypeLib GUID.", "Bad built application magic bytes.", "Specific driver is different from the specific driver associated with the Logical Name.", "There is no session opened to the class driver.", "Max Error", "MAX - Error with config objects", "MAX - Error loading configuration", "MAX - Group not supported"]
        # "Handle target timeout error here.\nWhen this JKISM could not get the sync-call response in time, this JKISM goes into this case."
        # "Handle mistyped state name (developer tool)"
        n40 = Format Into String(format string="Software Exception: Target could not finish the \"%s\" state in time." ("message"), error in=w157, w152) -> (resulting string=w160:string, error out=w159:errorcluster)  [unwired: 1 in]
        n41 = call <vilib>:"Error Cluster From Error Code.vi"("show call chain? (False)"=TRUE, "error in (no error)"=w159, "error message (\"\")"=w160, "error code (0)"=w161) -> ("error out"=w158:errorcluster)  [unwired: 5 in]
        n42 = call <vilib>:"Add State(s) to Queue__JKI_lib_State_Machine.vi"("State(s) in (\"\")"=w156) -> ("States Out"=w155:string)  [unwired: 14 in]
      }
      frame "Target Error" {
        w175 = 42 items=["No error", "Argument error", "Memory is full", "Out of zone", "End of file", "File already open", "Generic file I/O error", "File not found", "File permission error", "Disk is full", "Duplicate path", "Too many files open", "System feature not enabled", "Resource file not found", "Cannot add resource", "Resource not found", "Image not found", "Image memory error", "Pen does not exist", "Config type invalid", "Config token not found", "Config parse error", "Config memory error", "Bad external code format", "Bad external code offset", "External code not present", "Null window", "Destroy window error", "Null menu", "Print aborted", "Bad print record", "Print driver error", "Windows error during printing", "Memory error during printing", "Print dialog error", "Generic print error", "Invalid device refnum", "Device not found", "Device parameter error", "Device unit error", "Cannot open device", "Device call aborted", "Generic error", "Cancelled by user", "Object ID too low", "Object ID too high", "Object not in heap", "Unknown heap", "Unknown object (invalid DefProc)", "Unknown object (DefProc not in table)", "Message out of range", "Invalid (null) method", "Unknown message", "Manager call not supported", "Bad address", "Network operation in progress", "Network operation timed out", "Connection is busy", "Network attribute not supported", "Network error", "Address in use", "System out of memory", "Connection aborted", "Connection refused", "Not connected", "Already connected", "Connection closed", "Initialization error (interapplication manager)", "Bad occurrence", "Wait on unbound occurrence handler", "Occurrence queue overflow", "Datalog type conflict", "Unused", "Unrecognized type (interapplication manager)", "Memory corrupt", "Failed to make temporary DLL", "Old CIN version", "Drag socket not found", "Failed to load drop-object", "Failed to register OLE object", "Failed to release OLE object", "Format specifier type mismatch", "Unknown format specifier", "Too few format specifiers", "Too many format specifiers", "Scan failed", "Newer CIN version", "Error converting to variant", "Runtime menu error", "Password tampered", "Variant attribute not found", "Incompatible variant data type", "Event data is not available", "Event Store is not present", "Occurrence is not found", "Event Queue is not created", "Event info is not available", "Refnum passed is NULL", "Error retrieving Class GUID", "Error retrieving CoClass GUID", "Error retrieving TypeLib GUID.", "Bad built application magic bytes.", "Specific driver is different from the specific driver associated with the Logical Name.", "There is no session opened to the class driver.", "Max Error", "MAX - Error with config objects", "MAX - Error loading configuration", "MAX - Group not supported"]
        # "Handle target error here.\nWhen this JKISM try to communicate with an un-existed JKISM, this JKISM goes into this case."
        # "Handle mistyped state name (developer tool)"
        n43 = Format Into String(format string="Software Exception: Target \"%s\" does not exists." ("message"), error in=w171, w166) -> (resulting string=w174:string, error out=w173:errorcluster)  [unwired: 1 in]
        n44 = call <vilib>:"Error Cluster From Error Code.vi"("show call chain? (False)"=TRUE, "error in (no error)"=w173, "error message (\"\")"=w174, "error code (0)"=w175) -> ("error out"=w172:errorcluster)  [unwired: 5 in]
        n45 = call <vilib>:"Add State(s) to Queue__JKI_lib_State_Machine.vi"("State(s) in (\"\")"=w170) -> ("States Out"=w169:string)  [unwired: 14 in]
      }
      frame "Async Response", "Response" {
        # "Handle Async-call Response (\"Async Response\" for ->)"
        # "Handle Sync-call Response (\"Response\" for @)"
        # "After Message is excuted, JKISM+ goes to this state for recieve the response. \n    For Async Message(->), \"Async Response\" is used. This JKISM will goes to \"Async Message Posted\" immediately and recieve the \"Async Response\" after the callee finishes the message.\n    For Sync Message(@),  This JKISM will wait until the message is done and immidieatly goes to \"Response\""
      }
      frame "Async Message Posted" {
        # "Handle post action for async message (->)."
        # "After Async Message is posted (->), JKISM+ goes to this state for post-action. You can use Argument - State to tell which Async Message is called."
      }
      frame "Initialize Core Data" {
        # "Do not delete, rename, or modify this frame.\n(this is used to determine panel behavior on exit)"
        # "originally closed?"
        # "exe?"
        # "If panel starts closed or is an EXE, then close it when we exit"
        n46 = property class="VI"() -> ("FP.State"=w196:T1)  [unwired: 2 in, 2 out]
        n47 = property class="App"() -> ("App.Kind"=w201:T2)  [unwired: 2 in, 2 out]
        n48 = control-ref of="Current VI Reference"() -> (w197:refnum<vi>)
        n49 = Equal?(x=w196, y=T1."Closed" ("Front Panel Window:State")) -> (x = y?=w194:bool)
        n50 = Equal?(x=w201, y=T2."Run Time System" ("Application:Kind")) -> (x = y?=w199:bool)
        n51 = Or(x=w194, y=w199) -> (x .or. y?=w198:bool)
        n52 = Bundle By Name(cluster=w191, "Core.Current VI Reference"=w197, "Core.Close Panel on Exit?"=w198) -> (w190:T3)
        n53 = call <vilib>:"Add State(s) to Queue__JKI_lib_State_Machine.vi"("State(s) in (\"\")"=w204) -> ("States Out"=w203:string)  [unwired: 14 in]
      }
      frame "Exit" {
        # "Do not put any code in this frame.\n(No errors that occur here will be handled.)"
        n54 = call <vilib>:"Add State(s) to Queue__JKI_lib_State_Machine.vi"("State(s) in (\"\")"=w212) -> ("States Out"=w211:string)  [unwired: 14 in]
      }
      frame "---------- Data ----------" {
        # "Do not put any code in this frame.\n(It is a separator no-op. You can make a copy of this frame to create a new Data frame)"
        n55 = call <vilib>:"Add State(s) to Queue__JKI_lib_State_Machine.vi"("State(s) in (\"\")"=w219) -> ("States Out"=w218:string)  [unwired: 14 in]
      }
      frame "Data: Initialize" {
        w224 = T4 {"PIN"="", "First"="", "Last"="", "Amount"=""}  # Account Info
        w229 = T5 {"Current VI Reference"=refnum, "Close Panel on Exit?"=FALSE}  # Core
        # "do not delete - used by framework"
        # "Expand Bundle to add new data elements to shift register data."
        # "Data names and types of shift register data are defined by this bundle."
        # "Initialize the shift-register data, here.\n(data names are defined by what you wire into the bundle function)"
        n56 = call <vilib>:"Application Directory.vi"() -> ("Application Directory"=w227:path)
        n57 = Build Path(base path=w227, name or relative path="Accounts.txt") -> (appended path=w223:path)
        n58 = call-poly <vilib>:"Read Delimited Spreadsheet.vi"("file path (dialog if empty)"=w223, "delimiter (\\t)"="," ("delimiter (\\t)")) -> ("all rows"=w225:string[][])  [unwired: 8 in, 5 out]
        n59 = for {
          tunnel: w225 -> [w239] mode=indexing
          tunnel: [w234] -> w220 mode=indexing
          tunnel: w224 -> [w233]
          n60 = Index Array(array=w239) -> (element #1=w238:string, element #2=w237:string, element #3=w236:string, element #4=w235:string)  [unwired: 4 in]
          n61 = Bundle By Name(cluster=w233, "PIN"=w238, "First"=w237, "Last"=w236, "Amount"=w235) -> (w234:T4)
        }
        n62 = Bundle("Core"=w229) -> (w221:T3)  [unwired: 1 in]
        n63 = call <vilib>:"Add State(s) to Queue__JKI_lib_State_Machine.vi"("State(s) in (\"\")"=w232) -> ("States Out"=w231:string)  [unwired: 14 in]
      }
      frame "Data: Cleanup" {
        # "Cleanup any data and references, here.\n(this is called automatically, by the Macro: Exit)"
        n64 = Unbundle By Name(w242) -> ("Core.Current VI Reference"=w241:refnum<vi>)
        n65 = Close Reference(reference=w241, error in (no error)=w246) -> (error out=w245:errorcluster)
        n66 = call <vilib>:"Add State(s) to Queue__JKI_lib_State_Machine.vi"("State(s) in (\"\")"=w248) -> ("States Out"=w247:string)  [unwired: 14 in]
      }
      frame "---------- Events ----------" {
        # "Do not put any code in this frame.\n(It is a separator no-op. You can make a copy of this frame to create a new UI frame)"
        n67 = call <vilib>:"Add State(s) to Queue__JKI_lib_State_Machine.vi"("State(s) in (\"\")"=w255) -> ("States Out"=w254:string)  [unwired: 14 in]
      }
      frame "Events: Register" {
        # "Register message event to break Waiting in Event structure."
        n68 = call <userlib>:"JKISM++ Get New State Notifier Event.vi"("Name(\"\" to use uuid) in"=w260) -> ("Error out"=w258:errorcluster, "New State Notifier Event"=w259:refnum<user-event>)  [unwired: 9 in]
        n69 = register-events(w259) -> (reference out=w261:refnum<event-registration>)  [unwired: 2 in, 1 out]
      }
      frame "Events: Unregister" {
        n70 = Unregister For Events(event registration refnum=w266, error in=w270) -> (error out=w267:errorcluster)
      }
      frame "---------- UI ----------" {
        # "Do not put any code in this frame.\n(It is a separator no-op. You can make a copy of this frame to create a new UI frame)"
        n71 = call <vilib>:"Add State(s) to Queue__JKI_lib_State_Machine.vi"("State(s) in (\"\")"=w277) -> ("States Out"=w276:string)  [unwired: 14 in]
      }
      frame "UI: Initialize" {
        # "Initialize the User Interface, here.\n(this is called automatically, by the Macro: Init)"
        n72 = call <vilib>:"Add State(s) to Queue__JKI_lib_State_Machine.vi"("State(s) in (\"\")"=w284) -> ("States Out"=w283:string)  [unwired: 14 in]
      }
      frame "UI: Cursor Set" {
        # "Argument"
        # "Set and Unset Cursor Busy.\n(Usage: \"UI: Cursor Set >> Busy|Idle\")"
        n73 = case shown="\"Idle\", Default" w288 {
          tunnel: w290 -> [w295 w297]
          tunnel: [w294 w296] -> w289
          frame "Idle", Default {
            n74 = call <vilib>:"Unset Busy.vi"("error in (no error)"=w295) -> ("error out"=w294:errorcluster)  [unwired: 10 in]
          }
          frame "Busy" {
            n75 = call <vilib>:"Set Busy.vi"("error in (no error)"=w297) -> ("error out"=w296:errorcluster)  [unwired: 9 in, 1 out]
          }
        }
        n76 = call <vilib>:"Add State(s) to Queue__JKI_lib_State_Machine.vi"("State(s) in (\"\")"=w293) -> ("States Out"=w292:string)  [unwired: 14 in]
      }
      frame "UI: Front Panel State" {
        # "Argument"
        # "Set Front Panel Open or Closed\n(Usage: \"UI: Front Panel State >> Open|Close\")"
        n77 = Unbundle By Name(w299) -> ("Core.Current VI Reference"=w303:refnum<vi>)
        n78 = case shown="\"Open\", \"Standard\", Default" w302 {
          tunnel: w305 -> [w313 w326 w337 w349 w361]
          tunnel: [w314 w327 w338 w350 w362] -> w304
          tunnel: w303 -> [_ _ _ _ _]
          frame "Open", "Standard", Default {
            w308 = T1."Standard" ("State")
            n79 = property class="VI"(error in=w313) -> (reference out=w311:refnum<vi>, error out=w312:errorcluster, "FP.State"=w310:T1)  [unwired: 1 in]
            n80 = Not Equal?(x=w310, y=w308) -> (x != y?=w309:bool)
            n81 = case shown="False" w309 {
              tunnel: [w318 w320] -> w314
              tunnel: w312 -> [w317 w320]
              tunnel: w311 -> [w316 _]
              tunnel: w308 -> [w315 _]
              frame True {
                n82 = invoke class="VI" method="FP.Open"(reference=w316, error in=w317, "Activate"=TRUE, "State"=w315) -> (error out=w318:errorcluster)  [unwired: 1 in, 4 out]
              }
              frame False {
              }
            }
          }
          frame "Close", "Closed" {
            n83 = property class="VI"(error in=w326) -> (reference out=w324:refnum<vi>, error out=w325:errorcluster, "FP.State"=w322:T1)  [unwired: 1 in]
            n84 = Not Equal?(x=w322, y=T1."Closed" ("Front Panel Window:State")) -> (x != y?=w321:bool)
            n85 = case shown="True" w321 {
              tunnel: [w328 w331] -> w327
              tunnel: w325 -> [w328 w330]
              tunnel: w324 -> [_ w329]
              frame False {
              }
              frame True {
                n86 = invoke class="VI" method="FP.Close"(reference=w329, error in=w330) -> (error out=w331:errorcluster)  [unwired: 1 in, 2 out]
              }
            }
          }
          frame "Hidden", "Hide" {
            w332 = T1."Hidden" ("State")
            n87 = property class="VI"(error in=w337) -> (reference out=w335:refnum<vi>, error out=w336:errorcluster, "FP.State"=w334:T1)  [unwired: 1 in]
            n88 = Not Equal?(x=w334, y=w332) -> (x != y?=w333:bool)
            n89 = case shown="True" w333 {
              tunnel: [w342 w343] -> w338
              tunnel: w336 -> [w341 w343]
              tunnel: w335 -> [w340 _]
              tunnel: w332 -> [w339 _]
              frame True {
                n90 = invoke class="VI" method="FP.Open"(reference=w340, error in=w341, "State"=w339) -> (error out=w342:errorcluster)  [unwired: 2 in, 4 out]
              }
              frame False {
              }
            }
          }
          frame "Minimize", "Minimized" {
            w344 = T1."Minimized" ("State")
            n91 = property class="VI"(error in=w349) -> (reference out=w347:refnum<vi>, error out=w348:errorcluster, "FP.State"=w346:T1)  [unwired: 1 in]
            n92 = Not Equal?(x=w346, y=w344) -> (x != y?=w345:bool)
            n93 = case shown="True" w345 {
              tunnel: [w354 w355] -> w350
              tunnel: w348 -> [w353 w355]
              tunnel: w347 -> [w352 _]
              tunnel: w344 -> [w351 _]
              frame True {
                n94 = invoke class="VI" method="FP.Open"(reference=w352, error in=w353, "State"=w351) -> (error out=w354:errorcluster)  [unwired: 2 in, 4 out]
              }
              frame False {
              }
            }
          }
          frame "Maximize", "Maximized" {
            w356 = T1."Maximized" ("State")
            n95 = property class="VI"(error in=w361) -> (reference out=w359:refnum<vi>, error out=w360:errorcluster, "FP.State"=w358:T1)  [unwired: 1 in]
            n96 = Not Equal?(x=w358, y=w356) -> (x != y?=w357:bool)
            n97 = case shown="True" w357 {
              tunnel: [w366 w367] -> w362
              tunnel: w360 -> [w365 w367]
              tunnel: w359 -> [w364 _]
              tunnel: w356 -> [w363 _]
              frame True {
                n98 = invoke class="VI" method="FP.Open"(reference=w364, error in=w365, "State"=w363) -> (error out=w366:errorcluster)  [unwired: 2 in, 4 out]
              }
              frame False {
              }
            }
          }
        }
        n99 = call <vilib>:"Add State(s) to Queue__JKI_lib_State_Machine.vi"("State(s) in (\"\")"=w307) -> ("States Out"=w306:string)  [unwired: 14 in]
      }
      frame "---------- Macro ----------" {
        # "Do not put any code in this frame.\n(It is a separator no-op. You can make a copy of this frame to create a new Macro frame)"
        n100 = call <vilib>:"Add State(s) to Queue__JKI_lib_State_Machine.vi"("State(s) in (\"\")"=w374) -> ("States Out"=w373:string)  [unwired: 14 in]
      }
      frame "Macro: Initialize" {
        w378 = "Data: Initialize\nInitialize Core Data\nEvents: Register\nUI: Initialize\nUI: Front Panel State >> Open"  # Data: Initialize Initialize Core Data Events: Register UI: Initialize UI: Front Panel State >> Open
        # "Initialization Macro\n(This is called once, when the VI starts)"
        n101 = call <vilib>:"Add State(s) to Queue__JKI_lib_State_Machine.vi"("State(s) in Front (\"\")"=w378, "State(s) in (\"\")"=w382) -> ("States Out"=w381:string)  [unwired: 13 in]
      }
      frame "Macro: Exit" {
        # "Exit Macro\n(This is called once, when the VI exits)"
        n102 = Unbundle By Name(w385) -> ("Core.Close Panel on Exit?"=w384:bool)
        n103 = Select(t="UI: Front Panel State >> Close", s=w384, f="") -> (s? t:f=w390:string)
        n104 = call <vilib>:"Add State(s) to Queue__JKI_lib_State_Machine.vi"("State(s) in (\"\")"=w390, "State(s) at Back (\"\")"="Data: Cleanup\nEvents: Unregister\nExit") -> ("States Out"=w388:string)  [unwired: 13 in]
        n105 = call <vilib>:"Add State(s) to Queue__JKI_lib_State_Machine.vi"("State(s) in Front (\"\")"=w388, "State(s) in (\"\")"=w395) -> ("States Out"=w394:string)  [unwired: 13 in]
      }
      frame "---------- Action ----------" {
        # "Template Separator\n(You can make a copy of, or modify, this frame)"
        n106 = call <vilib>:"Add State(s) to Queue__JKI_lib_State_Machine.vi"("State(s) in (\"\")"=w402) -> ("States Out"=w401:string)  [unwired: 14 in]
      }
      frame "Action: PostErr" {
        # "Copy/Rename this case for your own API"
        n107 = call <userlib>:"JKISM++ Check If Module Exists.vi"("Error in"=w405, "JKISM Name"="Error Handler" ("Dest Module (\"\")")) -> ("Error out"=w404:errorcluster, "Exist?"=w407:bool)  [unwired: 7 in, 1 out]
        n108 = case shown="True" w407 {
          tunnel: w406 -> [_ w423]
          tunnel: ["Macro: Exit" w416] -> w403
          frame False {
          }
          frame True {
            n109 = call <userlib>:"Build State String with Arguments++.vi"("State"="Error Handler", "Arguments (\"\")"=w423, "Dest Module (\"\")"="Error Handler" ("Dest Module (\"\")"), "Sync-Call(@) T By Default/Async-Call(->) F"=FALSE) -> ("State with Arguments"=w417:string)  [unwired: 11 in]
            n110 = Concatenate Strings(w417, "\r", "Macro: Exit") -> (w416:string)
          }
        }
        n111 = call <vilib>:"Add State(s) to Queue__JKI_lib_State_Machine.vi"("State(s) in (\"\")"=w410, "State(s) at Back (\"\")"=w403) -> ("States Out"=w409:string)  [unwired: 13 in]
      }
      frame "Action: Find Account" {
        # "假设字符串形式John,Doe,12345"
        # "找到返回HxStr（布尔）"
        # "找到的话输出名字，找不到输出空"
        # "Found?"
        # "Template Separator\n(You can make a copy of, or modify, this frame)"
        n112 = Match Pattern(string=w428, regular expression=",") -> (before substring=w427:string, after substring=w430:string)  [unwired: 1 in, 2 out]
        n113 = Match Pattern(string=w430, regular expression=",") -> (before substring=w426:string, after substring=w425:string)  [unwired: 1 in, 2 out]
        n114 = for {
          tunnel: [w452] -> w438
          tunnel: w439 -> [w456] mode=indexing
          tunnel: [w450] -> w433
          tunnel: [w449] -> w432
          tunnel: w427 -> [w448]
          tunnel: w426 -> [w447]
          tunnel: w425 -> [w446]
          stop <- w452 stop-if-true
          n115 = Unbundle By Name(w456) -> ("First"=w450:string, "Last"=w449:string, "PIN"=w451:string)
          n116 = Equal?(x=w448, y=w450) -> (x = y?=w455:bool)
          n117 = Equal?(x=w447, y=w449) -> (x = y?=w454:bool)
          n118 = Equal?(x=w446, y=w451) -> (x = y?=w453:bool)
          n119 = Compound Arithmetic op=AND(w455, w454, w453) -> (w452:bool)
        }
        "Find Account?" <- w438
        n120 = call <vilib>:"Space Constant.vi"() -> ("String"=w442:string)
        n121 = Concatenate Strings(w433, w442, w432) -> (w441:string)
        n122 = call <userlib>:"JKISM++ Convert Data to HexStr.vi"("Variant"=w438) -> ("HEX String (0-9,A-F)"=w424:string)  [unwired: 8 in]
        n123 = Select(t=w441, s=w438, f="") -> (s? t:f=→"若有需要返回用户姓名，后面也可以接到esponse上":string)
        n124 = call <vilib>:"Add State(s) to Queue__JKI_lib_State_Machine.vi"("State(s) in (\"\")"=w435) -> ("States Out"=w436:string)  [unwired: 14 in]
      }
      frame "Action: Update Balance" {
        # "假设字符串形蔱,12345,1500"
        # "并无加减操作"
        # "只改变了指定PIN的数据，然后写入"
        # "HEX String 数值变动，Set Value"
        # "Search for record"
        # "Update \"Amount\" field"
        # "Your code here.\n(You can make a copy of, or modify, this frame)"
        n125 = Match Pattern(string=w460, regular expression=",") -> (before substring=w458:string, after substring=w457:string)  [unwired: 1 in, 2 out]
        n126 = for {
          tunnel: w468 -> [w478] mode=indexing
          tunnel: [w480] -> _
          tunnel: [w479] -> w467
          tunnel: [w478] -> w469
          tunnel: w458 -> [w477]
          i -> [w479]
          stop <- w480 stop-if-true
          n127 = Unbundle By Name(w478) -> ("PIN"=w481:string)
          n128 = Equal?(x=w477, y=w481) -> (x = y?=w480:bool)
        }
        n129 = Bundle By Name(cluster=w469, "Amount"=w457) -> (w470:T4)
        n130 = Replace Array Subset(array=w468, new element=w470, index=w467) -> (w462:T6)
        n131 = for {
          tunnel: w462 -> [w476] mode=indexing
          tunnel: [w475] -> w466 mode=indexing
          n132 = Cluster To Array(cluster=w476) -> (array=w475:string[])
        }
        n133 = call-poly <vilib>:"Write Delimited Spreadsheet.vi"("file path (dialog if empty)"=w463, "2D data"=w466, "append to file? (new file:F)"=FALSE, "delimiter (\\t)"="," ("delimiter (\\t)")) -> ("error out"=w461:errorcluster)  [unwired: 10 in, 1 out]
        n134 = call <vilib>:"Add State(s) to Queue__JKI_lib_State_Machine.vi"("State(s) in (\"\")"=w474) -> ("States Out"=w473:string)  [unwired: 14 in]
      }
      frame "Action: Get Balance" {
        # "12345"
        # "返回余额"
        # "数据应该来源于其他模块，假设以此种形式"
        # "Template Separator\n(You can make a copy of, or modify, this frame)"
        n135 = for {
          tunnel: w486 -> [w497] mode=indexing
          tunnel: w485 -> [w495]
          tunnel: [w494] -> _
          tunnel: [w493] -> w484
          stop <- w494 stop-if-true
          n136 = Unbundle By Name(w497) -> ("PIN"=w496:string, "Amount"=w493:string)
          n137 = Equal?(x=w495, y=w496) -> (x = y?=w494:bool)
        }
        n138 = Decimal String To Number(string=w484) -> (number=w482:i32)  [unwired: 2 in, 1 out]
        "Balance" <- w482
        n139 = call <userlib>:"JKISM++ Convert Data to HexStr.vi"("Variant"=w482) -> ("HEX String (0-9,A-F)"=w483:string)  [unwired: 8 in]
        n140 = call <vilib>:"Add State(s) to Queue__JKI_lib_State_Machine.vi"("State(s) in (\"\")"=w492) -> ("States Out"=w491:string)  [unwired: 14 in]
      }
    }
  }
